vi "CAN_Interface_Motor.vi"(8 "error in (no error)":errorcluster) -> (0 "error out":errorcluster)   [LabVIEW 2018]
uses:
  <vilib>/Platform/TimedLoop/XDataNode/timing_clust.ctl
  <vilib>/Platform/TimedLoop/XDataNode/nitl_modes.ctl
  <vilib>/Platform/TimedLoop/XDataNode/wakeup.ctl
  Type_Def/Master_DataControl.ctl
  Type_Def/TypeDef_cRIODatas.ctl
  Type_Def/Type_Def IMUDatas.ctl
  Type_Def/TypeDef_BMSDatas.ctl
  Type_Def/TypeDef_BMSStatuss.ctl
  Type_Def/TypeDef FixedMotorData.ctl
  Type_Def/Type_Def Actuator Controls.ctl
  Type_Def/Type_Def ControlState.ctl
  <vilib>/CANopenLib/CANOPEN.llb/CANopen Interface Create.vi
  <vilib>/CANopenLib/CANOPEN.llb/CANopen Heartbeat Create.vi
  <vilib>/CANopenLib/CANOPEN.llb/CANopen SDO Create.vi
  <vilib>/CANopenLib/CANOPEN.llb/CANopen SDO Write [I8].vi
  <vilib>/CANopenLib/CANOPEN.llb/CANopen SDO Write [I32].vi
  <vilib>/CANopenLib/CANOPEN.llb/CANopen SDO Write [U16].vi
  <vilib>/CANopenLib/CANOPEN.llb/CANopen SDO Read [I32].vi
  <vilib>/CANopenLib/CANOPEN.llb/CANopen SDO Read [U8].vi
  <vilib>/CANopenLib/CANOPEN.llb/CANopen SDO Close.vi
  <vilib>/CANopenLib/CANOPEN.llb/CANopen Interface Close.vi
  <vilib>/Platform/TimedLoop/XDataNode/XDataNode.xnode
  <vilib>/Platform/TimedLoop/XDataNode/XDNodeRunTimeDep.lvlib
panel:
  in  "Consumer Time (ms)":u16=10
  in  "period (ms)":i64=10
  in  "node-ID":u8=1 min=1 max=127 step=1
  in  "baud rate":u32(ring)=2 items=["1 Mbit/s"=0, "800 kbit/s"=1, "500 kbit/s"=2, "250 kbit/s"=3, "125 kbit/s"=4, "50 kbit/s"=6, "20 kbit/s"=7, "10 kbit/s"=8]
  in  "CANopen interface":u32(ring) items=["CANopen01", "CANopen02", "CANopen03", "CANopen04", "CANopen05", "CANopen06", "CANopen07", "CANopen08", "CANopen09", "CANopen10", "CANopen11", "CANopen12", "CANopen13", "CANopen14", "CANopen15", "CANopen16", "CANopen17", "CANopen18", "CANopen19", "CANopen20", "CANopen21", "CANopen22", "CANopen23", "CANopen24", "CANopen25", "CANopen26", "CANopen27", "CANopen28", "CANopen29", "CANopen30", "CANopen31", "CANopen32"]
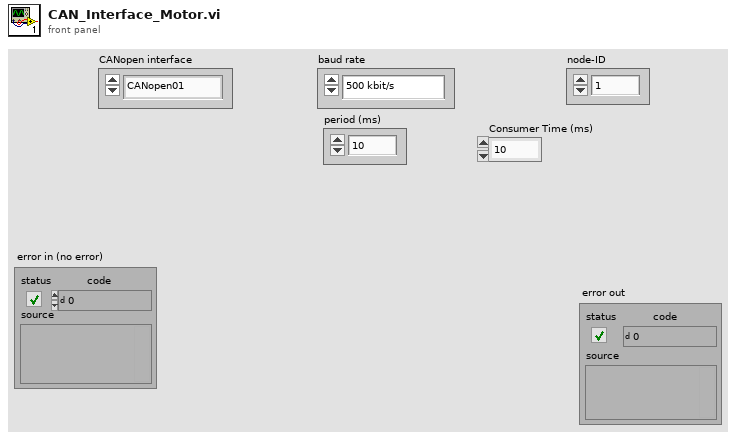
[diagram p1: front panel]
types:
  T1 = typedef "XDNodeRunTimeDep.lvlib/timing_clust.ctl" = cluster{"Expected End [f-1]":u64, "Actual End [f-1]":u64, "Finished Late? [f-1]":bool, "Expected End [i-1]":u64, "Actual End [i-1]":u64, "Finished Late? [i-1]":bool, "Expected Start [i]":u64, "Actual Start [i]":u64, "Expected Start [f]":u64, "Actual Start [f]":u64, "Source Name":string, "Structure Name":string, "Period":i64, "Deadline":i64, "Offset":i64, "Start":i64, "Priority":i32, "Timeout":i32, "Mode":T2, "Wakeup Reason":T3, "Error":errorcluster, "Source Type":string, "Secondary Source Type":string, "Global End Time":u64, "Global Start Time":u64, "Frame Duration":u64, "Iteration Duration":u64, "Assigned CPU":i32, "I/O Scan Engine Mode":u32}
  T2 = typedef "XDNodeRunTimeDep.lvlib/nitl_modes.ctl" = enum32{"No Change", "Process missed periods, maintain original phase", "Discard missed periods, maintain original phase", "Process missed periods, ignore original phase", "Discard missed periods, ignore original phase"}
  T3 = typedef "XDNodeRunTimeDep.lvlib/wakeup.ctl" = enum32{"Normal", "Aborted", "Asynchronous wakeup", "Timing source error", "Timed loop error", "Timeout"}
  T4 = typedef "Type_Def ControlState.ctl" = enum16{"Blank", "Systems Check", "Idle", "Ready", "Pushing", "CrawlingPrecharge", "Braking", "Fault", "Boot Up", "Crawling", "Shutdown", "Service Push", "Service Wait", "Vent", "Precharge"}
  T5 = typedef "Master_DataControl.ctl" = cluster{"cRIO Data":T6, "IMU Data":T7, "BMS Data":T8, "Motor Data":T10}
  T6 = typedef "TypeDef_cRIODatas.ctl" = cluster{"HallEffect Right (cm)":dbl, "HallEffect Left (cm)":dbl, "Optical Sensor 1 (V)":dbl, "Optical Sensor 2 (V)":dbl, "24V Voltage  (V)":dbl, "24V Current (A)":dbl, "Contactor H1 Continuity":dbl, "Contactor L1 Continuity ":dbl, "Contactor H2 Continuity":dbl, "Contactor L2 Continuity ":dbl, "Brake PT(psig)":dbl, "Pump PT (psig)":dbl, "24V Temp   (C)":dbl, "Tank PT(psig) ":dbl, "ABS Pressure 1 (psig)":dbl, "ABS Pressure 2 (psig) ":dbl, "Displacement (ft)":dbl, "Velocity (ft/s)":dbl, "Time (ms)":dbl, "PV 1 Temp (C)":dbl, "PV2 Temp (C)":dbl}
  T7 = typedef "Type_Def IMUDatas.ctl" = cluster{"y acceleration (g)":dbl, "Pressure (psia)":dbl, "Temperature (C)":dbl}
  T8 = typedef "TypeDef_BMSDatas.ctl" = cluster{"Pack 1 Current (A)":dbl, "Pack 1 Voltage (V)":dbl, "Pack 1 Highest Temperature(C)":dbl, "BmsStatus1":T9, "Pack 2 Current (A)":dbl, "Pack 2 Voltage (V) ":dbl, "Pack 2 Highest Temperature(C) ":dbl, "BmsStatus 2":T9, "Pack 1 Cell Array (V)":dbl[], "Pack 2 Cell Array (V)":dbl[], "Pack 1 Lowest Temperature (C)":dbl, "Pack 1 Average Temperature (C)":dbl, "Pack 2 Average Temperature (C)":dbl, "Pack 2 Lowest Temperature (C)":dbl}
  T9 = typedef "TypeDef_BMSStatuss.ctl" = cluster{"isFault":bool, "isolationMonitoring":bool}
  T10 = typedef "TypeDef FixedMotorData.ctl" = cluster{" Velocity (RPM)":dbl, " MotorTemp(C)":dbl, " ControlTemp(C)":dbl, " DcLinkVolt(V)":dbl, " ErrorCode":dbl, "IsAlive":bool, "motorStatus":cluster{"isReady":bool, "isOn":bool, "isOperEn":bool, "isFault":bool, "isVoltEn":bool, "targetReached":bool, "isWarning":bool}, "motorControllerState":u16}
  T11 = typedef "Type_Def Actuator Controls.ctl" = cluster{"Reverse ":bool, "Precharge Ctrl":bool, "Pump Ctrl":bool, "24 VDC Ctr":bool, "Vent Solenoid":bool, "Brake Solenoid":bool, "EMCY  Brake Solenoid":bool, "Digital Out 7B ":bool, "Forward Ctrl":bool, " Contact H2":bool, "Contact L2":bool, "LED RED":bool, "LED GREEN":bool, " Digital Out 7A":bool, " Contact H1":bool, "Contact L1":bool}
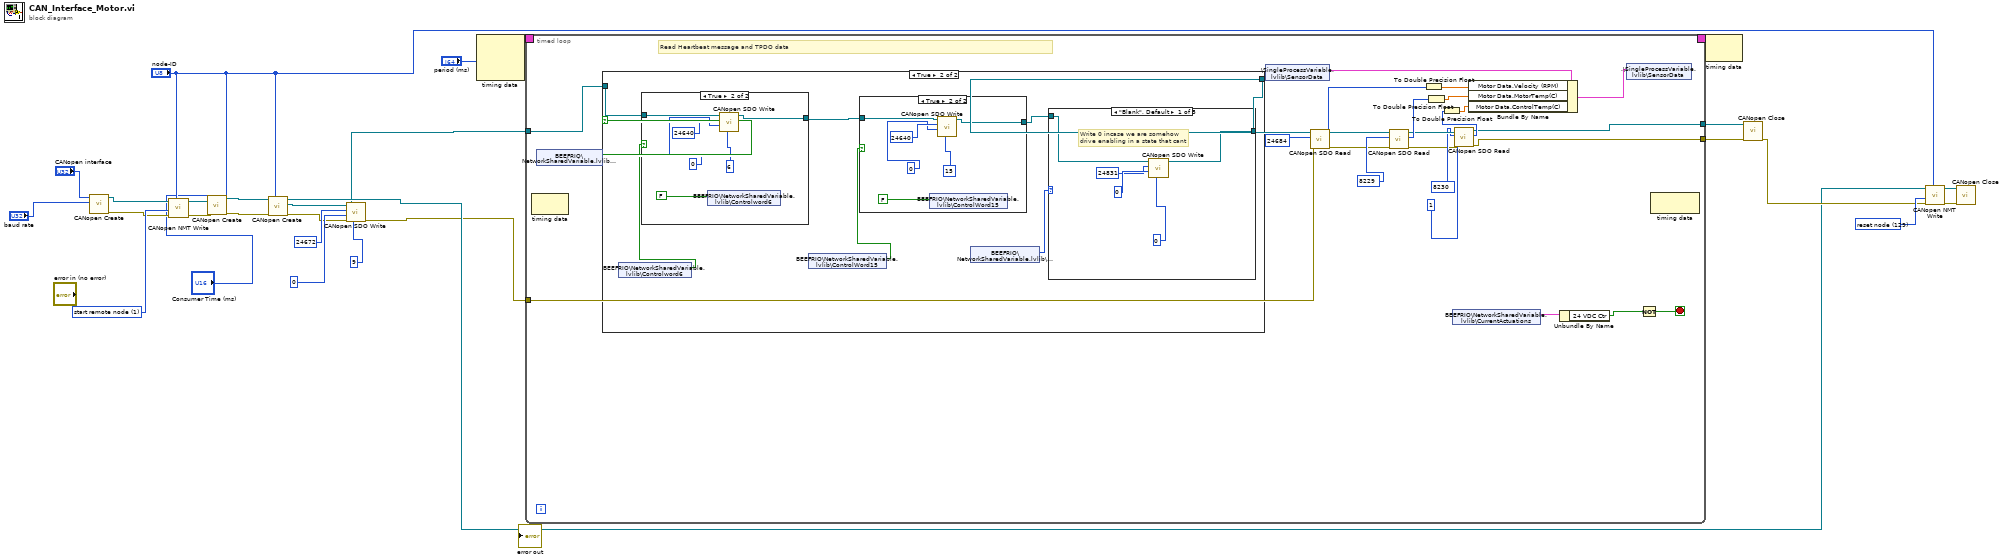
[diagram p0: block diagram]
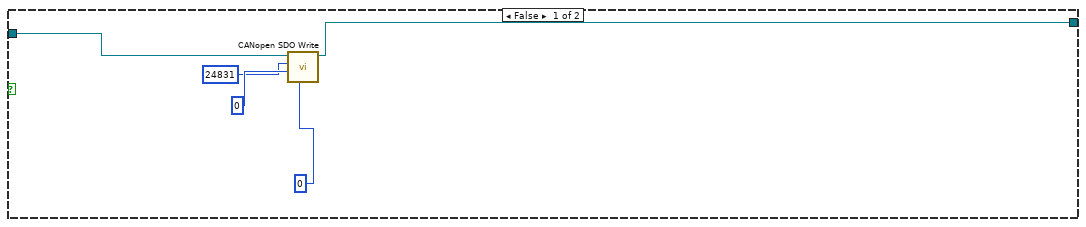
[diagram p2: hidden frame]
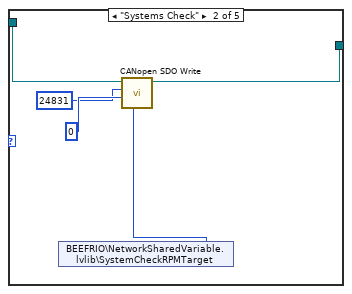
[diagram p5: hidden frame]
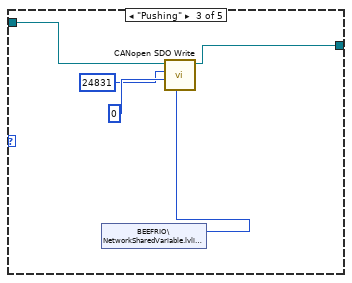
[diagram p6: hidden frame]
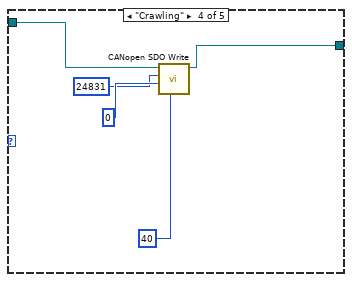
[diagram p7: hidden frame]
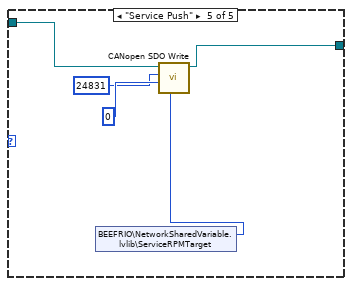
[diagram p8: hidden frame]
diagram:
  w18 = u16 1 items=["start remote node"=1, "stop remote node"=2, "enter pre-operational"=128, "reset node"=129, "reset communication"=130] ("command")
  w24 = u16 129 items=["start remote node"=1, "stop remote node"=2, "enter pre-operational"=128, "reset node"=129, "reset communication"=130] ("command")
  n1 = call-poly <vilib>:"CANopen Create.vi"("baud rate"="baud rate", "interface name"="CANopen interface") -> ("error out"=w17:errorcluster, "interface object out"=w19:refnum<k20>)  [unwired: 8 in]
  n2 = call <vilib>:"CANopen NMT Write.vi"("node-ID (0)"="node-ID", "error in (no error)"=w17, "command"=w18, "interface object in"=w19) -> ("error out"=w15:errorcluster, "interface object out"=w13:refnum<k20>)  [unwired: 6 in]
  n3 = call-poly <vilib>:"CANopen Create.vi"("node-ID"="node-ID", "error in (no error)"=w15, "consumer time [ms]"="Consumer Time (ms)", "interface object in"=w13) -> ("error out"=w14:errorcluster, "interface object out"=w12:refnum<k20>)  [unwired: 5 in, 1 out]
  n4 = call-poly <vilib>:"CANopen Create.vi"("node-ID"="node-ID", "error in (no error)"=w14, "interface object in"=w12) -> ("error out"=w5:errorcluster, "SDO object out"=w9:refnum<k20>, "interface object out"=w3:refnum<k20>)  [unwired: 6 in]
  n5 = call-poly <vilib>:"CANopen SDO Write.vi"("I8 data"=i8 9, "error in (no error)"=w5, "object sub-index (0)"=u8 0, "object index"=u16 24672, "SDO object in"=w9) -> ("error out"=w2:errorcluster, "SDO object out"=w1:refnum<k20>)  [unwired: 4 in, 1 out]
  n6 = node-c288("period (ms)") -> (w28:T1)  [unwired: 2 in]
  n7 = timed-loop {
    timing: w28 -> [_]
    timing-out: [_] -> w27
    tunnel: w1 -> [w53]
    tunnel: [w35] -> w16
    tunnel: w2 -> [w32]
    tunnel: [w29] -> w4
    stop <- w50 stop-if-true
    # "Read Heartbeat message and TPDO data"
    n8 = node-c288() -> ()  [unwired: 1 in, 1 out]
    n9 = shared-variable "BEEFRIO\\NetworkSharedVariable.lvlib\\driveEnable"() -> (w49:bool)  [unwired: 1 in, 1 out]
    n10 = case shown="True" w49 {
      tunnel: w53 -> [w55 w63]
      tunnel: [w54 w65] -> w48
      frame False {
        n11 = call-poly <vilib>:"CANopen SDO Write.vi"("I32 data"=u8 0 ("object sub-index (0)"), "object sub-index (0)"=u8 0, "object index"=u16 24831, "SDO object in"=w55) -> ("SDO object out"=w54:refnum<k20>)  [unwired: 5 in, 2 out]
      }
      frame True {
        n12 = shared-variable "BEEFRIO\\NetworkSharedVariable.lvlib\\Controlword6"() -> (w62:bool)  [unwired: 1 in, 1 out]
        n13 = case shown="True" w62 {
          tunnel: w63 -> [w73 w77]
          tunnel: [w73 w76] -> w60
          frame False {
          }
          frame True {
            n14 = shared-variable "BEEFRIO\\NetworkSharedVariable.lvlib\\Controlword6"(FALSE) -> ()  [unwired: 1 in, 1 out]
            n15 = call-poly <vilib>:"CANopen SDO Write.vi"("U16 data"=u16 6, "object sub-index (0)"=u8 0, "object index"=u16 24640, "SDO object in"=w77) -> ("SDO object out"=w76:refnum<k20>)  [unwired: 5 in, 2 out]
          }
        }
        n16 = shared-variable "BEEFRIO\\NetworkSharedVariable.lvlib\\ControlWord15"() -> (w61:bool)  [unwired: 1 in, 1 out]
        n17 = case shown="True" w61 {
          tunnel: [w66 w70] -> w59
          tunnel: w60 -> [w66 w68]
          frame False {
          }
          frame True {
            n18 = shared-variable "BEEFRIO\\NetworkSharedVariable.lvlib\\ControlWord15"(FALSE) -> ()  [unwired: 1 in, 1 out]
            n19 = call-poly <vilib>:"CANopen SDO Write.vi"("U16 data"=u16 15, "object sub-index (0)"=u8 0, "object index"=u16 24640, "SDO object in"=w68) -> ("SDO object out"=w70:refnum<k20>)  [unwired: 5 in, 2 out]
          }
        }
        n20 = shared-variable "BEEFRIO\\NetworkSharedVariable.lvlib\\CurrentState"() -> (w64:T4)  [unwired: 1 in, 1 out]
        n21 = case shown="\"Blank\", Default" w64 {
          tunnel: w59 -> [w82 w87 w91 w97 w101]
          tunnel: [w80 w86 w90 w95 w100] -> w65
          frame "Blank", Default {
            # "Write 0 incase we are somehow\ndrive enabling in a state that cant"
            n22 = call-poly <vilib>:"CANopen SDO Write.vi"("I32 data"=0 ("object sub-index (0)"), "object sub-index (0)"=u8 0, "object index"=u16 24831, "SDO object in"=w82) -> ("SDO object out"=w80:refnum<k20>)  [unwired: 5 in, 2 out]
          }
          frame "Systems Check" {
            n23 = shared-variable "BEEFRIO\\NetworkSharedVariable.lvlib\\SystemCheckRPMTarget"() -> (w85:i32)  [unwired: 1 in, 1 out]
            n24 = call-poly <vilib>:"CANopen SDO Write.vi"("I32 data"=w85, "object sub-index (0)"=u8 0, "object index"=u16 24831, "SDO object in"=w87) -> ("SDO object out"=w86:refnum<k20>)  [unwired: 5 in, 2 out]
          }
          frame "Pushing" {
            n25 = shared-variable "BEEFRIO\\NetworkSharedVariable.lvlib\\driveTarget"() -> (w92:i32)  [unwired: 1 in, 1 out]
            n26 = call-poly <vilib>:"CANopen SDO Write.vi"("I32 data"=w92, "object sub-index (0)"=u8 0, "object index"=u16 24831, "SDO object in"=w91) -> ("SDO object out"=w90:refnum<k20>)  [unwired: 5 in, 2 out]
          }
          frame "Crawling" {
            n27 = call-poly <vilib>:"CANopen SDO Write.vi"("I32 data"=40, "object sub-index (0)"=u8 0, "object index"=u16 24831, "SDO object in"=w97) -> ("SDO object out"=w95:refnum<k20>)  [unwired: 5 in, 2 out]
          }
          frame "Service Push" {
            n28 = shared-variable "BEEFRIO\\NetworkSharedVariable.lvlib\\ServiceRPMTarget"() -> (w102:i32)  [unwired: 1 in, 1 out]
            n29 = call-poly <vilib>:"CANopen SDO Write.vi"("I32 data"=w102, "object sub-index (0)"=u8 0, "object index"=u16 24831, "SDO object in"=w101) -> ("SDO object out"=w100:refnum<k20>)  [unwired: 5 in, 2 out]
          }
        }
      }
    }
    n30 = shared-variable ".\\SingleProcessVariable.lvlib\\SensorData"() -> (w46:T5)  [unwired: 1 in, 1 out]
    n31 = call-poly <vilib>:"CANopen SDO Read.vi"("error in (no error)"=w32, "object index"=u16 24684, "SDO object in"=w48) -> ("error out"=w31:errorcluster, "I32 data"=w45:i32, "SDO object out"=w43:refnum<k20>)  [unwired: 5 in, 1 out]
    n32 = call-poly <vilib>:"CANopen SDO Read.vi"("error in (no error)"=w31, "object index"=u16 8229, "SDO object in"=w43) -> ("error out"=w30:errorcluster, "U8 data"=w40:u8, "SDO object out"=w39:refnum<k20>)  [unwired: 5 in, 1 out]
    n33 = To Double Precision Float(number=w45) -> (double precision float=w44:dbl)
    n34 = To Double Precision Float(number=w40) -> (double precision float=w41:dbl)
    n35 = shared-variable "BEEFRIO\\NetworkSharedVariable.lvlib\\CurrentActuations"() -> (w52:T11)  [unwired: 1 in, 1 out]
    n36 = call-poly <vilib>:"CANopen SDO Read.vi"("error in (no error)"=w30, "object sub-index (0)"=1, "object index"=u16 8230, "SDO object in"=w39) -> ("error out"=w29:errorcluster, "U8 data"=w38:u8, "SDO object out"=w35:refnum<k20>)  [unwired: 4 in, 1 out]
    n37 = To Double Precision Float(number=w38) -> (double precision float=w37:dbl)
    n38 = Bundle By Name(cluster=w46, "Motor Data.Velocity (RPM)"=w44, "Motor Data.MotorTemp(C)"=w41, "Motor Data.ControlTemp(C)"=w37) -> (w36:T5)
    n39 = Unbundle By Name(w52) -> ("24 VDC Ctr"=w51:bool)
    n40 = shared-variable ".\\SingleProcessVariable.lvlib\\SensorData"(w36) -> ()  [unwired: 1 in, 1 out]
    n41 = Not(x=w51) -> (.not. x?=w50:bool)
    n42 = node-c288() -> ()  [unwired: 1 in, 1 out]
  }
  n43 = node-c288(w27) -> ()  [unwired: 1 out]
  n44 = call-poly <vilib>:"CANopen Close.vi"("error in (no error)"=w4, "SDO object in"=w16) -> ("error out"=w23:errorcluster)  [unwired: 9 in]
  n45 = call <vilib>:"CANopen NMT Write.vi"("node-ID (0)"="node-ID", "error in (no error)"=w23, "command"=w24, "interface object in"=w3) -> ("error out"=w26:errorcluster, "interface object out"=w25:refnum<k20>)  [unwired: 6 in]
  n46 = call-poly <vilib>:"CANopen Close.vi"("error in (no error)"=w26, "interface object in"=w25) -> ()  [unwired: 9 in, 1 out]
